vi "!_Read-Write_Setups.vi"(2 "Port Settings Array In":T1[](array[typedef]) {"flow control etc."."parity err byte" format="%.0x"; "flow control etc."."XON byte" format="%.0x"; "flow control etc."."XOFF byte" format="%.0x"; "data bits" min=5 max=8 step=1}, 3 "Setup Name":string, 4 "Mode":enum16{"Load serial setup", "Save serial setup"}(ring)) -> (0 "Port Settings Array Out":T1[](array[typedef]) {"flow control etc."."parity err byte" format="%.0x"; "flow control etc."."XON byte" format="%.0x"; "flow control etc."."XOFF byte" format="%.0x"; "data bits" min=5 max=8 step=1}, 1 "error unflattening":bool)   [LabVIEW 2022 SP3]
uses:
  Port_Params.ctl
  Anemometry/Anemometry Sub Vis/Globals/Constants_global.vi
  Serial_Logging_Global.vi
panel:
  out "readFlatstring":string
  out "writtenFlatstring":string
  out "readError":errorcluster
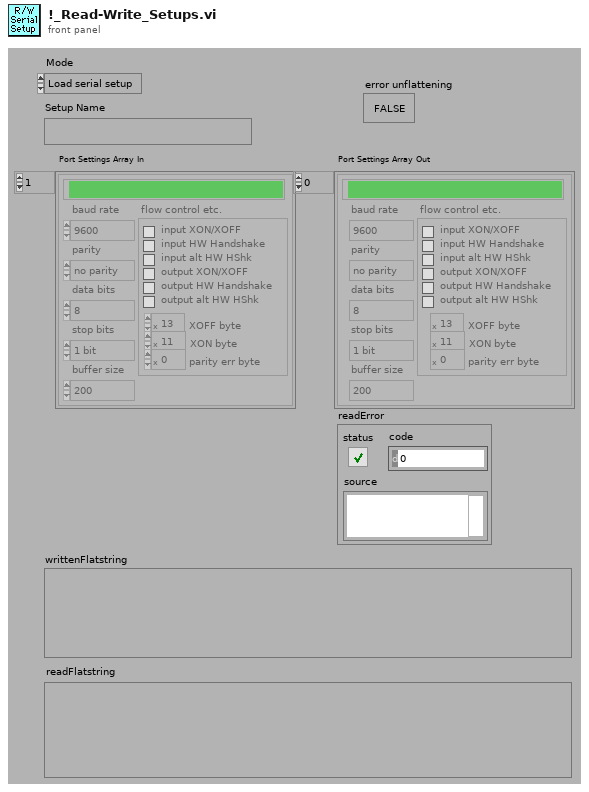
[diagram p1: front panel]
types:
  T1 = typedef "Port_Params.ctl" = cluster{"Name":string, "flow control etc.":cluster{"input XON/XOFF":bool, "input HW Handshake":bool, "input alt HW HShk":bool, "output XON/XOFF":bool, "output HW Handshake":bool, "output alt HW HShk":bool, "XOFF byte ":u8, "XON byte":u8, "parity err byte":u16}, "buffer size":u16, "baud rate":u32, "data bits":u16, "stop bits":enum16{"1 bit", "1.5 bits", "2 bits"}, "parity":enum16{"no parity", "odd parity", "even parity", "mark parity", "space parity"}}
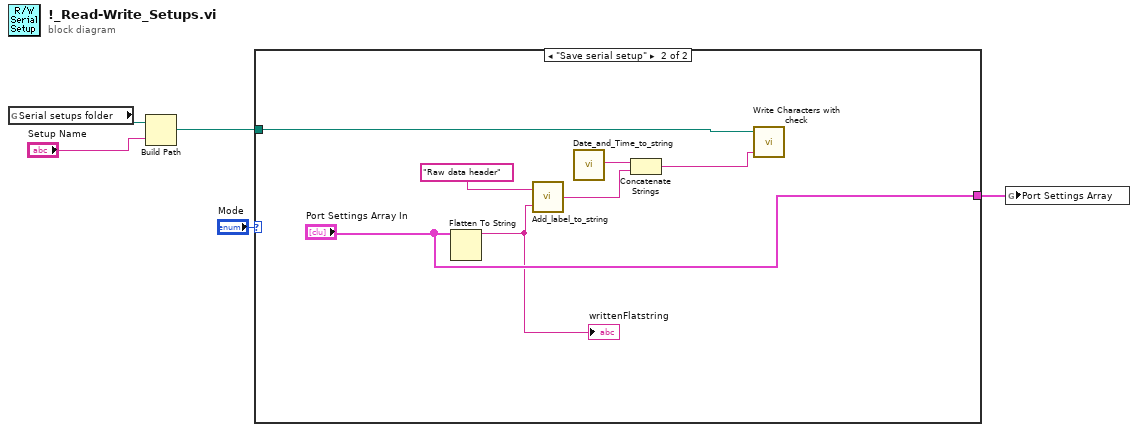
[diagram p0: block diagram]
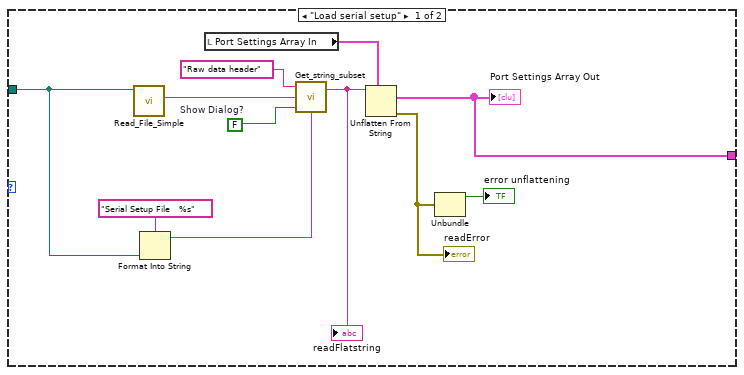
[diagram p2: hidden frame]
diagram:
  n1 = global read "Constants_global.vi" "Serial setups folder"() -> (w4:path)
  n2 = Build Path(base path=w4, name or relative path="Setup Name") -> (appended path=w3:path)
  n3 = case shown="\"Save serial setup\"" "Mode" {
    tunnel: w3 -> [w8 w18]
    tunnel: [w7 "Port Settings Array In"] -> w1
    frame "Load serial setup" {
      w12 = FALSE  # Show Dialog?
      n4 = call "Read_File_Simple.vi"("Filename"=w8) -> ("string"=w15:string)  [unwired: 2 in, 7 out]
      n5 = Format Into String(format string="Serial Setup File   %s", w8) -> (resulting string=w6:string)  [unwired: 2 in, 1 out]
      n6 = local read "Port Settings Array In"() -> (w11:T1[])
      n7 = call "Get_string_subset.vi"("String Name"=w6, "Show Dialog?"=w12, "String to split"=w15, "File Label"="Raw data header") -> ("Output string"=w14:string)  [unwired: 1 out]
      "readFlatstring" <- w14
      n8 = Unflatten From String(type=w11, binary string=w14) -> (value=w7:T1[], error out=w10:errorcluster)  [unwired: 1 in, 3 out]
      "Port Settings Array Out" <- w7
      "readError" <- w10
      n9 = Unbundle(w10) -> ("status"=→"error unflattening":bool)  [unwired: 2 out]
    }
    frame "Save serial setup" {
      n10 = Flatten To String(anything="Port Settings Array In") -> (data string=w19:string)  [unwired: 1 in, 4 out]
      "writtenFlatstring" <- w19
      n11 = call "Add_label_to_string.vi"("String to write"=w19, "File Label"="Raw data header") -> ("Output string"=w21:string)
      n12 = call "Date_and_Time_to_string.vi"() -> ("Date and time (spreadsheet)"=w22:string)  [unwired: 4 in, 1 out]
      n13 = Concatenate Strings(w22, w21) -> (w17:string)
      n14 = call "Write Characters with check.vi"("String to Write"=w17, "file (use dialog)"=w18) -> ()  [unwired: 2 in, 1 out]
    }
  }
  n15 = global write "Serial_Logging_Global.vi" "Port Settings Array"(w1) -> ()
